vi "Wave Memory Generator.vi"(8 "Scaling factor":dbl=1.0, 9 "Custom Triangular Signal (fal-ris)":dbl[](array[numeric])=[2047.0, 2034.0, 2022.0, 2010.0, 1998.0, 1986.0, 1974.0, 1962.0, 1949.0, 1937.0, 1925.0, 1913.0, 1901.0, 1889.0, 1877.0, 1866.0, 1854.0, 1842.0, 1830.0, 1818.0, 1806.0, 1794.0, 1782.0, 1771.0, 1759.0, 1747.0, 1735.0, 1724.0, 1712.0, 1700.0, 1689.0, 1677.0, 1665.0, 1654.0, 1642.0, 1631.0, 1619.0, 1608.0, 1596.0, 1584.0, 1573.0, 1562.0, 1550.0, 1539.0, 1527.0, 1516.0, 1504.0, 1493.0, 1482.0, 1470.0, 1459.0, 1448.0, 1437.0, 1425.0, 1414.0, 1403.0, 1392.0, 1381.0, 1369.0, 1358.0, 1347.0, 1336.0, 1325.0, 1314.0, 1303.0, 1292.0, 1281.0, 1270.0, 1259.0, 1248.0, 1237.0, 1226.0, 1215.0, 1204.0, 1193.0, 1182.0, 1172.0, 1161.0, 1150.0, 1139.0, 1128.0, 1118.0, 1107.0, 1096.0, 1086.0, 1075.0, 1064.0, 1054.0, 1043.0, 1032.0, 1022.0, 1011.0, 1001.0, 990.0, 980.0, 969.0, 959.0, 948.0, 938.0, 927.0, 917.0, 907.0, 896.0, 886.0, 876.0, 865.0, 855.0, 845.0, 834.0, 824.0, 814.0, 804.0, 794.0, 783.0, 773.0, 763.0, 753.0, 743.0, 733.0, 723.0, 713.0, 703.0, 693.0, 683.0, 673.0, 663.0, 653.0, 643.0, 633.0, 623.0, 613.0, 603.0, 594.0, 584.0, 574.0, 564.0, 555.0, 545.0, 535.0, 525.0, 516.0, 506.0, 496.0, 487.0, 477.0, 468.0, 458.0, 448.0, 439.0, 429.0, 420.0, 410.0, 401.0, 392.0, 382.0, 373.0, 363.0, 354.0, 345.0, 335.0, 326.0, 317.0, 307.0, 298.0, 289.0, 280.0, 270.0, 261.0, 252.0, 243.0, 234.0, 225.0, 216.0, 206.0, 197.0, 188.0, 179.0, 170.0, 161.0, 152.0, 143.0, 134.0, 126.0, 117.0, 108.0, 99.0, 90.0, 81.0, 72.0, 64.0, 55.0, 46.0, 37.0, 29.0, 20.0, 11.0, 2.0, -6.0, -15.0, -23.0, -32.0, -41.0, -49.0, -58.0, -66.0, -75.0, -83.0, -92.0, -100.0, -109.0, -117.0, -126.0, -134.0, -143.0, -151.0, -159.0, -168.0, -176.0, -184.0, -193.0, -201.0, -209.0, -218.0, -226.0, -234.0, -242.0, -251.0, -259.0, -267.0, -275.0, -283.0, -291.0, -300.0, -308.0, -316.0, -324.0, -332.0, -340.0, -348.0, -356.0, -364.0, -372.0, -380.0, -388.0, -396.0, -404.0, -412.0, -420.0, -428.0, -436.0, -444.0, -451.0, -459.0, -467.0, -475.0, -483.0, -490.0, -498.0, -506.0, -513.0, -521.0, -528.0, -536.0, -544.0, -551.0, -559.0, -566.0, -573.0, -581.0, -588.0, -595.0, -603.0, -610.0, -617.0, -624.0, -631.0, -638.0, -645.0, -652.0, -659.0, -666.0, -673.0, -680.0, -687.0, -693.0, -700.0, -707.0, -713.0, -720.0, -726.0, -733.0, -739.0, -746.0, -752.0, -758.0, -765.0, -771.0, -777.0, -783.0, -789.0, -795.0, -801.0, -807.0, -813.0, -818.0, -824.0, -830.0, -836.0, -841.0, -847.0, -852.0, -858.0, -863.0, -869.0, -874.0, -880.0, -885.0, -890.0, -896.0, -901.0, -906.0, -911.0, -917.0, -922.0, -927.0, -932.0, -937.0, -942.0, -947.0, -952.0, -957.0, -962.0, -967.0, -972.0, -977.0, -982.0, -987.0, -992.0, -997.0, -1002.0, -1007.0, -1012.0, -1016.0, -1021.0, -1026.0, -1031.0, -1036.0, -1041.0, -1045.0, -1050.0, -1055.0, -1060.0, -1064.0, -1069.0, -1074.0, -1079.0, -1083.0, -1088.0, -1093.0, -1097.0, -1102.0, -1107.0, -1111.0, -1116.0, -1121.0, -1125.0, -1130.0, -1134.0, -1139.0, -1144.0, -1148.0, -1153.0, -1157.0, -1162.0, -1166.0, -1171.0, -1175.0, -1180.0, -1184.0, -1188.0, -1193.0, -1197.0, -1202.0, -1206.0, -1210.0, -1215.0, -1219.0, -1223.0, -1228.0, -1232.0, -1236.0, -1240.0, -1245.0, -1249.0, -1253.0, -1257.0, -1262.0, -1266.0, -1270.0, -1274.0, -1278.0, -1282.0, -1286.0, -1291.0, -1295.0, -1299.0, -1303.0, -1307.0, -1311.0, -1315.0, -1319.0, -1323.0, -1327.0, -1331.0, -1335.0, -1339.0, -1343.0, -1346.0, -1350.0, -1354.0, -1358.0, -1362.0, -1366.0, -1370.0, -1374.0, -1377.0, -1381.0, -1385.0, -1389.0, -1393.0, -1396.0, -1400.0, -1404.0, -1408.0, -1411.0, -1415.0, -1419.0, -1422.0, -1426.0, -1430.0, -1433.0, -1437.0, -1441.0, -1444.0, -1448.0, -1452.0, -1455.0, -1459.0, -1462.0, -1466.0, -1470.0, -1473.0, -1477.0, -1480.0, -1484.0, -1488.0, -1491.0, -1495.0, -1498.0, -1502.0, -1505.0, -1509.0, -1513.0, -1516.0, -1520.0, -1523.0, -1527.0, -1530.0, -1534.0, -1538.0, -1541.0, -1545.0, -1548.0, -1552.0, -1555.0, -1559.0, -1563.0, -1566.0, -1570.0, -1573.0, -1577.0, -1581.0, -1584.0, -1588.0, -1591.0, -1595.0, -1599.0, -1602.0, -1606.0, -1609.0, -1613.0, -1616.0, -1620.0, -1624.0, -1627.0, -1631.0, -1634.0, -1638.0, -1641.0, -1645.0, -1648.0, -1652.0, -1655.0, -1659.0, -1662.0, -1666.0, -1669.0, -1673.0, -1676.0, -1680.0, -1683.0, -1686.0, -1690.0, -1693.0, -1697.0, -1700.0, -1703.0, -1707.0, -1710.0, -1713.0, -1717.0, -1720.0, -1723.0, -1727.0, -1730.0, -1733.0, -1736.0, -1740.0, -1743.0, -1746.0, -1749.0, -1752.0, -1756.0, -1759.0, -1762.0, -1765.0, -1768.0, -1772.0, -1775.0, -1778.0, -1781.0, -1784.0, -1787.0, -1791.0, -1794.0, -1797.0, -1800.0, -1803.0, -1806.0, -1809.0, -1813.0, -1816.0, -1819.0, -1822.0, -1825.0, -1828.0, -1831.0, -1835.0, -1838.0, -1841.0, -1844.0, -1847.0, -1850.0, -1853.0, -1857.0, -1860.0, -1863.0, -1866.0, -1869.0, -1872.0, -1876.0, -1879.0, -1882.0, -1885.0, -1888.0, -1891.0, -1895.0, -1898.0, -1901.0, -1904.0, -1907.0, -1910.0, -1914.0, -1917.0, -1920.0, -1923.0, -1926.0, -1929.0, -1933.0, -1936.0, -1939.0, -1942.0, -1945.0, -1949.0, -1952.0, -1955.0, -1958.0, -1961.0, -1965.0, -1968.0, -1971.0, -1974.0, -1977.0, -1981.0, -1984.0, -1987.0, -1990.0, -1994.0, -1997.0, -2000.0, -2003.0, -2006.0, -2010.0, -2013.0, -2016.0, -2019.0, -2023.0, -2026.0, -2029.0, -2032.0, -2036.0, -2039.0, -2042.0, -2045.0, -2048.0, -2048.0, -2036.0, -2024.0, -2012.0, -1999.0, -1987.0, -1975.0, -1963.0, -1951.0, -1939.0, -1926.0, -1914.0, -1902.0, -1890.0, -1878.0, -1866.0, -1854.0, -1842.0, -1831.0, -1819.0, -1807.0, -1795.0, -1783.0, -1771.0, -1760.0, -1748.0, -1736.0, -1725.0, -1713.0, -1701.0, -1690.0, -1678.0, -1667.0, -1655.0, -1644.0, -1632.0, -1621.0, -1609.0, -1598.0, -1587.0, -1575.0, -1564.0, -1553.0, -1542.0, -1530.0, -1519.0, -1508.0, -1497.0, -1486.0, -1475.0, -1463.0, -1452.0, -1441.0, -1430.0, -1419.0, -1408.0, -1397.0, -1387.0, -1376.0, -1365.0, -1354.0, -1343.0, -1332.0, -1322.0, -1311.0, -1300.0, -1290.0, -1279.0, -1268.0, -1258.0, -1247.0, -1237.0, -1226.0, -1216.0, -1205.0, -1195.0, -1184.0, -1174.0, -1163.0, -1153.0, -1143.0, -1133.0, -1122.0, -1112.0, -1102.0, -1092.0, -1081.0, -1071.0, -1061.0, -1051.0, -1041.0, -1031.0, -1021.0, -1011.0, -1001.0, -991.0, -981.0, -971.0, -961.0, -952.0, -942.0, -932.0, -922.0, -912.0, -903.0, -893.0, -883.0, -874.0, -864.0, -855.0, -845.0, -835.0, -826.0, -816.0, -807.0, -798.0, -788.0, -779.0, -769.0, -760.0, -751.0, -742.0, -732.0, -723.0, -714.0, -705.0, -696.0, -686.0, -677.0, -668.0, -659.0, -650.0, -641.0, -632.0, -623.0, -614.0, -605.0, -596.0, -588.0, -579.0, -570.0, -561.0, -552.0, -544.0, -535.0, -526.0, -518.0, -509.0, -501.0, -492.0, -483.0, -475.0, -466.0, -458.0, -449.0, -441.0, -433.0, -424.0, -416.0, -408.0, -399.0, -391.0, -383.0, -375.0, -366.0, -358.0, -350.0, -342.0, -334.0, -326.0, -318.0, -310.0, -302.0, -294.0, -286.0, -278.0, -270.0, -262.0, -254.0, -247.0, -239.0, -231.0, -223.0, -216.0, -208.0, -200.0, -193.0, -185.0, -177.0, -170.0, -162.0, -155.0, -147.0, -140.0, -132.0, -125.0, -117.0, -110.0, -102.0, -95.0, -87.0, -80.0, -73.0, -65.0, -58.0, -50.0, -43.0, -36.0, -28.0, -21.0, -13.0, -6.0, 1.0, 9.0, 16.0, 24.0, 31.0, 39.0, 46.0, 54.0, 61.0, 69.0, 76.0, 84.0, 92.0, 99.0, 107.0, 115.0, 122.0, 130.0, 138.0, 146.0, 153.0, 161.0, 169.0, 177.0, 185.0, 193.0, 201.0, 210.0, 218.0, 226.0, 234.0, 242.0, 251.0, 259.0, 267.0, 276.0, 284.0, 292.0, 301.0, 309.0, 318.0, 326.0, 335.0, 343.0, 351.0, 360.0, 368.0, 376.0, 385.0, 393.0, 401.0, 410.0, 418.0, 426.0, 434.0, 442.0, 450.0, 458.0, 466.0, 474.0, 482.0, 490.0, 498.0, 505.0, 513.0, 520.0, 528.0, 535.0, 542.0, 550.0, 557.0, 564.0, 570.0, 577.0, 584.0, 590.0, 596.0, 603.0, 609.0, 615.0, 621.0, 626.0, 632.0, 638.0, 643.0, 648.0, 653.0, 659.0, 664.0, 669.0, 673.0, 678.0, 683.0, 687.0, 692.0, 696.0, 701.0, 705.0, 709.0, 713.0, 717.0, 721.0, 725.0, 729.0, 733.0, 737.0, 741.0, 745.0, 748.0, 752.0, 756.0, 760.0, 763.0, 767.0, 770.0, 774.0, 778.0, 781.0, 785.0, 789.0, 792.0, 796.0, 800.0, 803.0, 807.0, 811.0, 815.0, 819.0, 823.0, 827.0, 831.0, 835.0, 839.0, 843.0, 847.0, 851.0, 855.0, 859.0, 863.0, 868.0, 872.0, 876.0, 880.0, 885.0, 889.0, 893.0, 898.0, 902.0, 906.0, 911.0, 915.0, 920.0, 924.0, 928.0, 933.0, 937.0, 941.0, 946.0, 950.0, 954.0, 959.0, 963.0, 967.0, 972.0, 976.0, 980.0, 984.0, 989.0, 993.0, 997.0, 1001.0, 1005.0, 1009.0, 1013.0, 1017.0, 1021.0, 1025.0, 1029.0, 1033.0, 1037.0, 1041.0, 1045.0, 1048.0, 1052.0, 1056.0, 1060.0, 1064.0, 1067.0, 1071.0, 1075.0, 1079.0, 1082.0, 1086.0, 1090.0, 1093.0, 1097.0, 1101.0, 1105.0, 1108.0, 1112.0, 1116.0, 1120.0, 1123.0, 1127.0, 1131.0, 1135.0, 1138.0, 1142.0, 1146.0, 1150.0, 1154.0, 1158.0, 1162.0, 1166.0, 1170.0, 1174.0, 1178.0, 1182.0, 1186.0, 1190.0, 1194.0, 1198.0, 1203.0, 1207.0, 1211.0, 1215.0, 1219.0, 1224.0, 1228.0, 1232.0, 1237.0, 1241.0, 1245.0, 1250.0, 1254.0, 1258.0, 1262.0, 1267.0, 1271.0, 1275.0, 1280.0, 1284.0, 1288.0, 1293.0, 1297.0, 1301.0, 1306.0, 1310.0, 1314.0, 1318.0, 1323.0, 1327.0, 1331.0, 1335.0, 1339.0, 1343.0, 1347.0, 1352.0, 1356.0, 1360.0, 1364.0, 1368.0, 1372.0, 1376.0, 1379.0, 1383.0, 1387.0, 1391.0, 1395.0, 1399.0, 1403.0, 1407.0, 1411.0, 1415.0, 1419.0, 1423.0, 1426.0, 1430.0, 1434.0, 1438.0, 1442.0, 1446.0, 1450.0, 1454.0, 1458.0, 1462.0, 1466.0, 1470.0, 1474.0, 1478.0, 1483.0, 1487.0, 1491.0, 1495.0, 1500.0, 1504.0, 1508.0, 1513.0, 1517.0, 1521.0, 1526.0, 1530.0, 1535.0, 1540.0, 1544.0, 1549.0, 1553.0, 1558.0, 1563.0, 1567.0, 1572.0, 1577.0, 1582.0, 1586.0, 1591.0, 1596.0, 1601.0, 1606.0, 1611.0, 1615.0, 1620.0, 1625.0, 1630.0, 1635.0, 1640.0, 1645.0, 1650.0, 1655.0, 1660.0, 1664.0, 1669.0, 1674.0, 1679.0, 1684.0, 1689.0, 1694.0, 1699.0, 1703.0, 1708.0, 1713.0, 1718.0, 1723.0, 1728.0, 1732.0, 1737.0, 1742.0, 1747.0, 1752.0, 1756.0, 1761.0, 1766.0, 1771.0, 1775.0, 1780.0, 1785.0, 1789.0, 1794.0, 1799.0, 1804.0, 1808.0, 1813.0, 1818.0, 1822.0, 1827.0, 1832.0, 1836.0, 1841.0, 1846.0, 1850.0, 1855.0, 1859.0, 1864.0, 1869.0, 1873.0, 1878.0, 1882.0, 1887.0, 1891.0, 1896.0, 1901.0, 1905.0, 1910.0, 1914.0, 1919.0, 1923.0, 1928.0, 1932.0, 1937.0, 1941.0, 1946.0, 1950.0, 1955.0, 1959.0, 1963.0, 1968.0, 1972.0, 1977.0, 1981.0, 1986.0, 1990.0, 1994.0, 1999.0, 2003.0, 2007.0, 2012.0, 2016.0, 2021.0, 2025.0, 2029.0, 2034.0, 2038.0, 2042.0, 2047.0], 11 "Triangolo dritto?":bool=TRUE) -> (0 "FXP Init Data Out":fxp<+/-,12,12>[](array[numeric]), 3 "Init Data Out":i64[](array[numeric]))   [LabVIEW 2014]
uses:
  <vilib>/Analysis/NI_AALPro.lvlib
  <vilib>/Analysis/NI_AALBase.lvlib
panel:
  out "Frequency (Hz)":dbl
  out "Init Data Out Graph":i64[](graph)
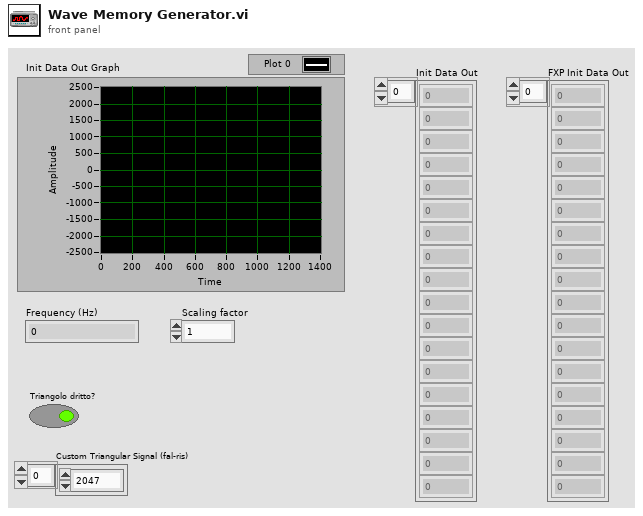
[diagram p1: front panel]
types:
  T1 = enum16{"sine", "cosine", "triangle", "square", "sawtooth", "increasing ramp", "decreasing ramp"}
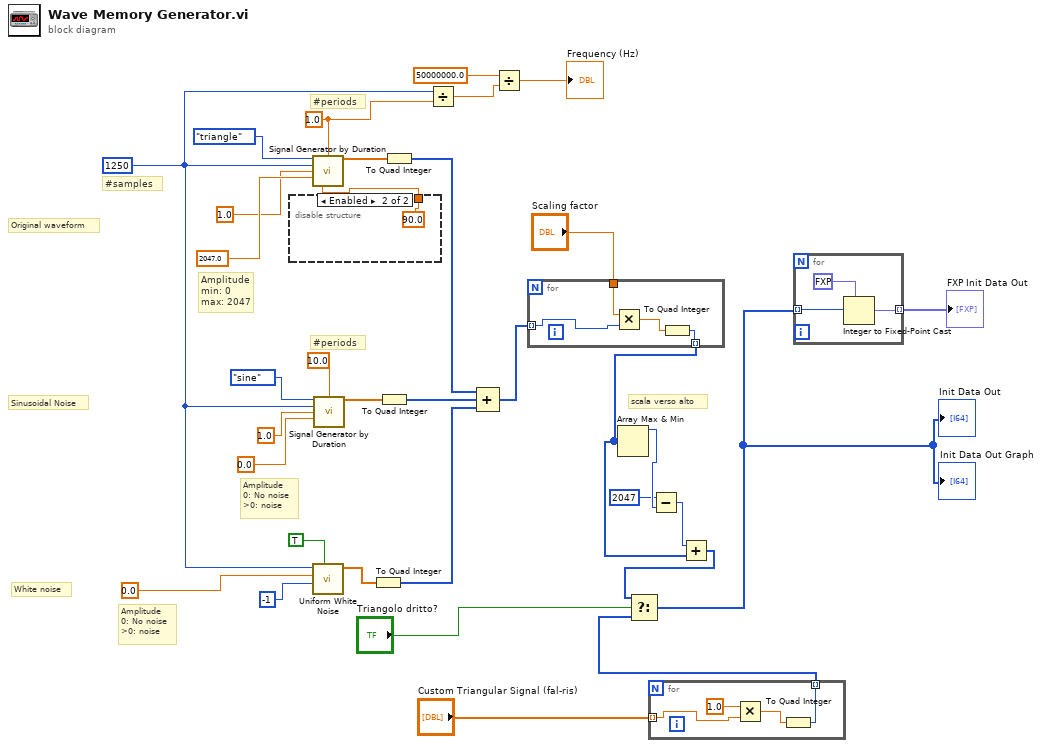
[diagram p0: block diagram]
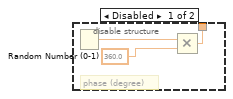
[diagram p2: hidden frame]
diagram:
  w15 = 1.0 ("duration")
  w16 = 1250 ("# of samples")
  # "scala verso alto"
  # "Amplitude\n0: No noise\n>0: noise"
  # "Original waveform"
  # "Sinusoidal Noise"
  # "White noise"
  # "#periods"
  # "Amplitude\n0: No noise\n>0: noise"
  # "#periods"
  # "Amplitude\nmin: 0\nmax: 2047"
  # "#samples"
  n1 = disable-structure shown="Enabled" {
    disable-tunnel: [w35 90.0 ("phase in")] -> w18
    frame Disabled {
      # "phase (degree)"
      n2 = Random Number (0-1)() -> (number: 0 to 1=w36:dbl)
      n3 = Multiply(x=w36, y=360.0) -> (x*y=w35:dbl)
    }
    frame Enabled {
    }
  }
  n4 = call <vilib>:"Signal Generator by Duration.vi"("signal type"=T1."triangle", "duration"=w15, "# of samples"=w16, "frequency"=1.0, "amplitude"=2047.0, "phase in"=w18) -> ("signal"=w20:dbl[])  [unwired: 6 in, 3 out]
  n5 = call <vilib>:"Uniform White Noise.vi"("initialize?"=TRUE, "seed"=-1, "amplitude"=0.0, "samples"=w16) -> ("uniform white noise"=w19:dbl[])  [unwired: 6 in, 1 out]
  n6 = call <vilib>:"Signal Generator by Duration.vi"("signal type"=T1."sine", "duration"=10.0, "# of samples"=w16, "frequency"=1.0, "amplitude"=0.0) -> ("signal"=w32:dbl[])  [unwired: 7 in, 3 out]
  n7 = To Quad Integer(1:w19) -> (0:w25:i64[])
  n8 = To Quad Integer(1:w32) -> (0:w27:i64[])
  n9 = To Quad Integer(1:w20) -> (0:w24:i64[])
  n10 = Divide(x=w16, y=w15) -> (x/y=w14:dbl)
  n11 = Compound Arithmetic op=ADD(w24, w27, w25) -> (w7:i64[])
  n12 = Divide(x=50000000.0, y=w14) -> (x/y=→"Frequency (Hz)":dbl)
  n13 = for {
    tunnel: w7 -> [w42] mode=indexing
    tunnel: [w40] -> w2 mode=indexing
    tunnel: "Scaling factor" -> [w39]
    n14 = Multiply(x=w39, y=w42) -> (x*y=w41:dbl)
    n15 = To Quad Integer(1:w41) -> (0:w40:i64)
  }
  n16 = Array Max & Min(array=w2) -> (max value=w5:i64)  [unwired: 3 out]
  n17 = for {
    tunnel: "Custom Triangular Signal (fal-ris)" -> [w45] mode=indexing
    tunnel: [w43] -> w10 mode=indexing
    n18 = Multiply(x=1.0, y=w45) -> (x*y=w44:dbl)
    n19 = To Quad Integer(1:w44) -> (0:w43:i64)
  }
  n20 = Subtract(x=i64 2047, y=w5) -> (x-y=w3:i64)
  n21 = Add(x=w3, y=w2) -> (x+y=w1:i64[])
  n22 = Select(t=w1, s="Triangolo dritto?", f=w10) -> (s? t:f=w11:i64[])
  "Init Data Out Graph" <- w11
  "Init Data Out" <- w11
  n23 = for {
    tunnel: w11 -> [w49] mode=indexing
    tunnel: [w47] -> w12 mode=indexing
    n24 = Integer to Fixed-Point Cast(fixed-point type=fxp<+/-,12,12> 0.0, integer=w49) -> (fixed-point=w47:fxp<+/-,12,12>)
  }
  "FXP Init Data Out" <- w12
